vi "OSF Upload File.vi"(6 "Append to\nLab Notebook":bool, 7 "timeout":dbl=60.0 format="%#_6ps", 8 "error in":errorcluster, 9 "Token":string, 10 "Node":string, 11 "File name":path=path "C:/Data/April_2019/042419/sp0006_042419.tdms") -> (0 "error out":errorcluster)   [LabVIEW 2021]
uses:
  <vilib>/httpClient/LabVIEWHTTPClient.lvlib
  <vilib>/httpClient/PUTFile.vi
  <vilib>/httpClient/PUTBuffer.vi
  <vilib>/Utility/TDMS File Viewer/NI_TDMS File Viewer.lvlib
panel:
  in  "View":bool
  out "Status":string
  in  "Upload":bool
  in  "Stop Button":bool
  in  "Export Type":enum16{"Text", "Markdown"}(ring)=enum."Markdown"
  out "Elapsed time":dbl format="%#_6ps"
  out "body 2":string
  out "body":string
  in  "OSF API URL":string="https://api.osf.io/v2/"
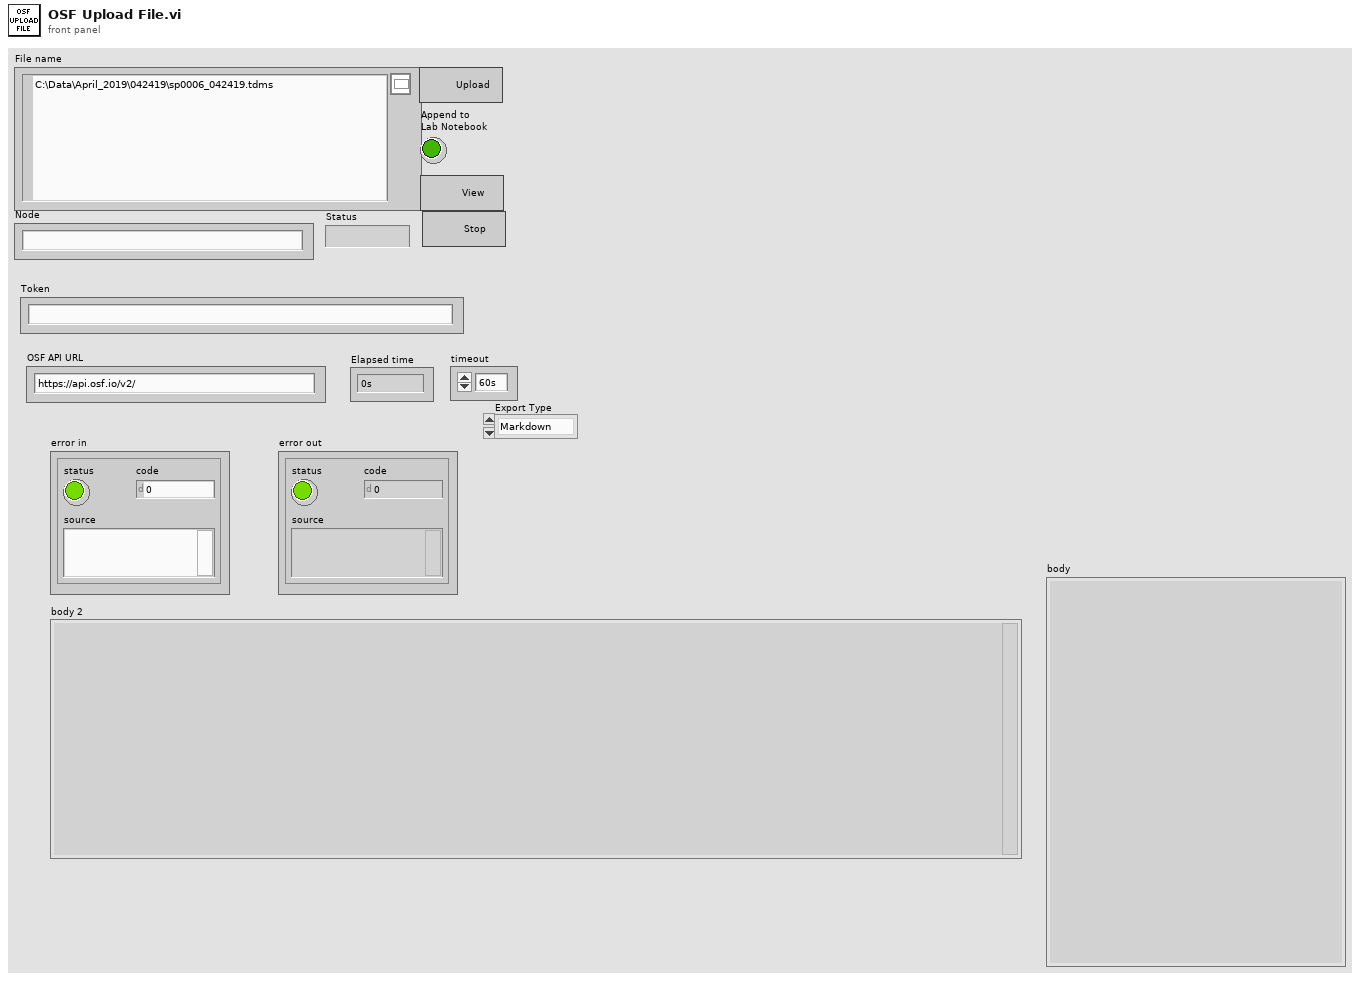
[diagram p1: front panel]
types:
  T1 = typedef "LabVIEWHTTPClient.lvlib/ClientHandle.ctl" = refnum<k1>
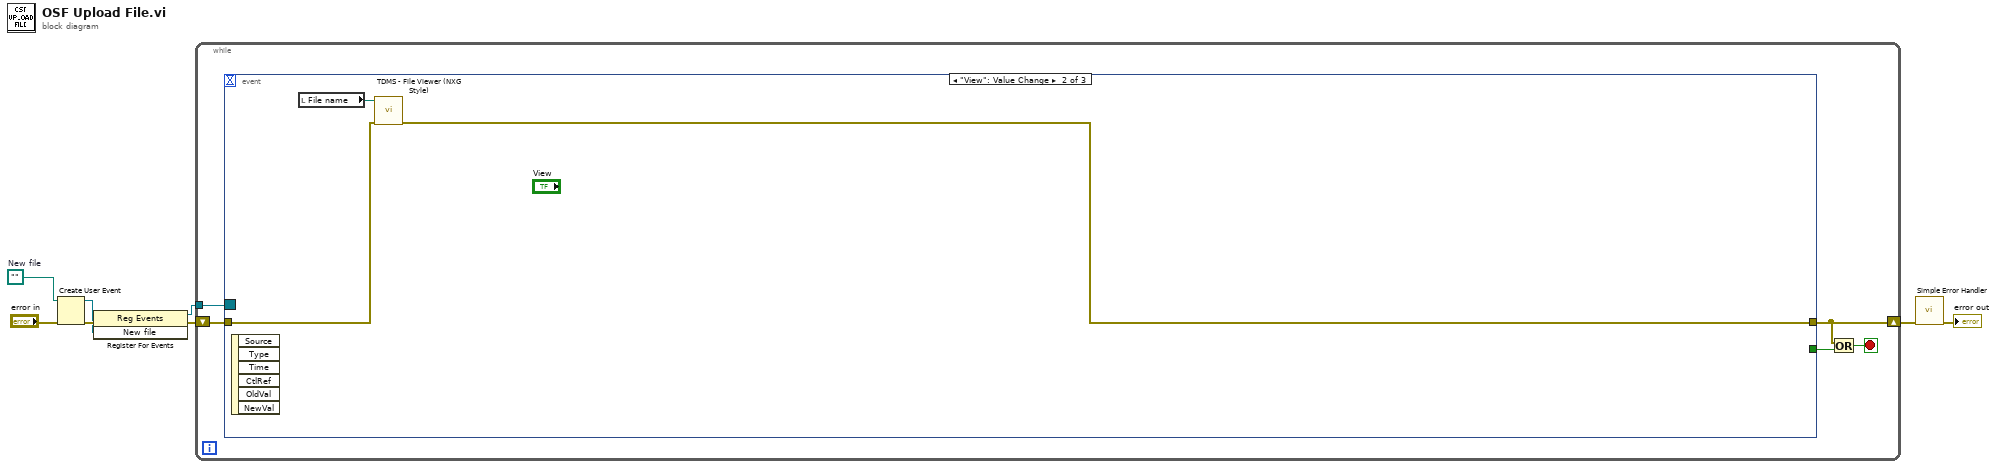
[diagram p0: block diagram]
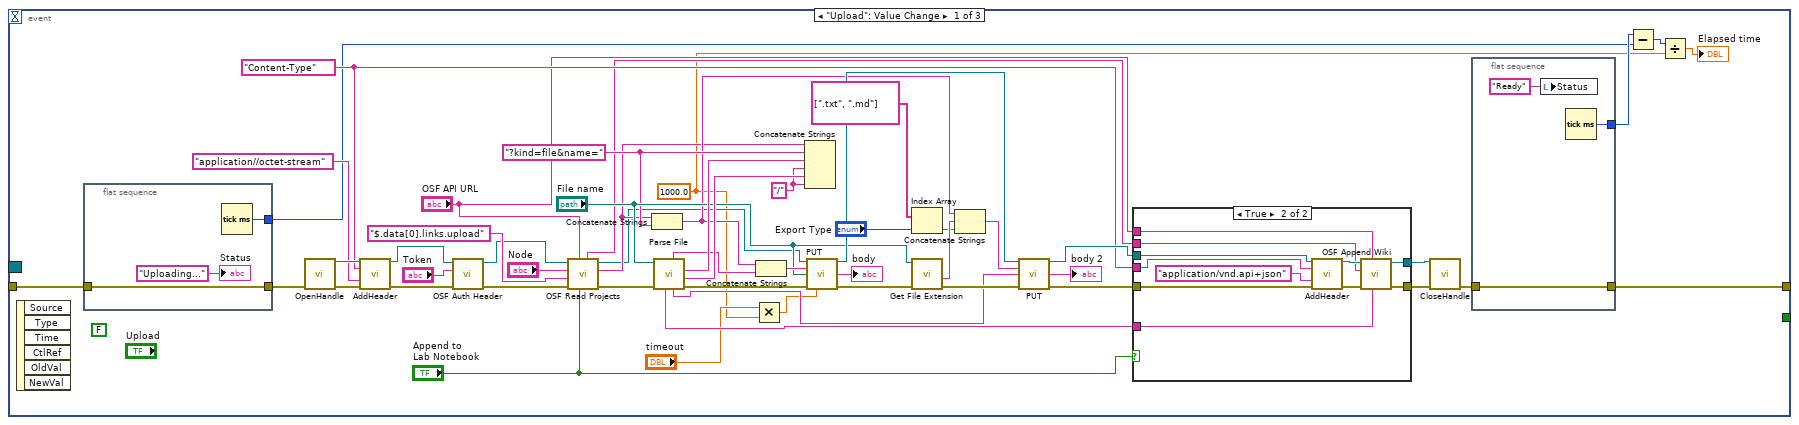
[diagram p2: hidden frame]
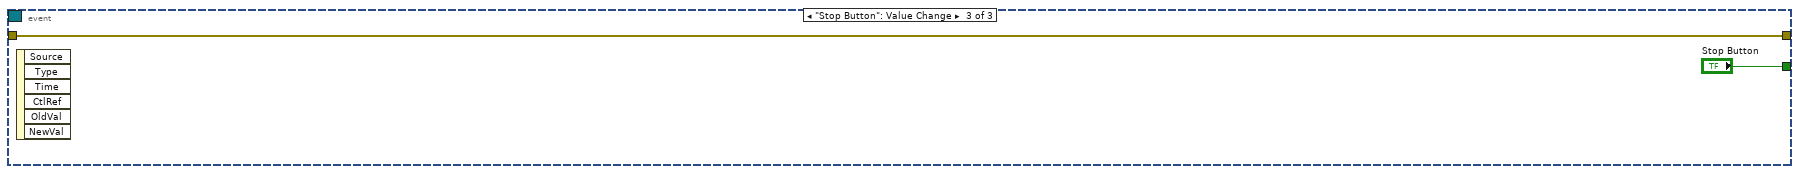
[diagram p4: hidden frame]
diagram:
  w3 = path ""  # New file
  n1 = Create User Event(user event datatype=w3, error in="error in") -> (user event=w1:refnum<user-event>, error out=w4:errorcluster)
  n2 = register-events(error in=w4, w1) -> (reference out=w5:refnum<event-registration>, error out=w6:errorcluster)  [unwired: 1 in]
  n3 = while {
    shift-right: [w10] -> w7
    shift-left: w6 -> [w13]
    tunnel: w5 -> [w9]
    stop <- w11 stop-if-true
    n4 = event shown="[1] \"View\": Value Change" {
      selector: w9 -> [_ _ _]
      dyn-events: _ -> [_ _ _]
      timeout: _ -> [_ _ _]
      tunnel: w13 -> [w25 w87 w89]
      tunnel: [w22 w86 w89] -> w10
      tunnel: [_ _ "Stop Button"] -> w12
      event "Upload": Value Change {
        (unwired) FALSE ("Top Button")
        w17 = 1000.0 ("y")
        w57 = "/" ("string")
        w46 = "?kind=file&name="
        w38 = "Content-Type" ("header")
        n5 = event-data() -> ()  [unwired: 1 in, 6 out]
        n6 = flat-sequence {
          tunnel: w25 -> [w72]
          tunnel: [w72] -> w24
          tunnel: [w71] -> w20
          frame #0 {
            n7 = Tick Count (ms)() -> (millisecond timer value=w71:u32)
            "Status" <- "Uploading..." ("Status")
          }
        }
        n8 = call <vilib>:"OpenHandle.vi"("error in (no error)"=w24) -> ("client handle out"=w66:T1, "error out"=w65:errorcluster)  [unwired: 13 in]
        n9 = call <vilib>:"AddHeader.vi"("client handle"=w66, "header"=w38, "value"="application//octet-stream", "error in (no error)"=w65) -> ("client handle out"=w61:T1, "error out"=w33:errorcluster)  [unwired: 10 in]
        n10 = call "OSF Auth Header.vi"("error in"=w33, "Token"="Token", "client handle"=w61) -> ("error out"=w30:errorcluster, "client handle out"=w31:T1)  [unwired: 7 in]
        n11 = call "OSF Read Projects.vi"("Read wikis"="Append to\nLab Notebook", "OSF API URL"="OSF API URL", "error in"=w30, "$Path or Item Name"="$.data[0].links.upload", "node"="Node", "client handle"=w31) -> ("error out"=w29:errorcluster, "Upload link"=w36:string, "client handle out"=w32:T1, "Wiki ID"=w35:string)  [unwired: 2 out]
        n12 = Concatenate Strings(w36, w46) -> (w45:string)
        n13 = call "Parse File.vi"("error in"=w29, "File name"="File name") -> ("error out"=w56:errorcluster, "Dir 2"=w58:string, "Dir 1"=w59:string, "metadata"=w41:string, "File name"=w42:string, "Lab notebook entry"=w28:string)  [unwired: 2 in, 2 out]
        n14 = Multiply(x="timeout", y=w17) -> (x*y=w26:dbl)
        n15 = Concatenate Strings(w45, w42) -> (w54:string)
        n16 = Concatenate Strings(w36, w46, w59, w57, w58, w57) -> ()  [unwired: 1 out]
        n17 = call-poly <vilib>:"PUT.vi"("client handle"=w32, "url"=w54, "file"="File name", "error in (no error)"=w56, "timeout (10000)"=w26) -> ("client handle out"=w55:T1, "body"=→"body":string, "error out"=w49:errorcluster)  [unwired: 7 in, 1 out]
        n18 = Index Array(array=string[] [".txt", ".md"], index="Export Type") -> (element=w16:string)
        n19 = call <vilib>:"Get File Extension.vi"("error in (no error)"=w49, "file"="File name") -> ("error out"=w48:errorcluster, "filename without extension"=w52:string)  [unwired: 5 in, 3 out]
        n20 = Concatenate Strings(w45, w52, w16) -> (w51:string)
        n21 = call-poly <vilib>:"PUT.vi"("client handle"=w55, "url"=w51, "buffer"=w41, "error in (no error)"=w48) -> ("client handle out"=w39:T1, "body"=→"body 2":string, "error out"=w40:errorcluster)  [unwired: 8 in, 1 out]
        n22 = case shown="True" "Append to\nLab Notebook" {
          tunnel: [w73 w85] -> w44
          tunnel: [w74 w84] -> w43
          tunnel: w28 -> [_ w83]
          tunnel: w40 -> [w74 w82]
          tunnel: w39 -> [w73 w80]
          tunnel: w38 -> [_ w78]
          tunnel: "OSF API URL" -> [_ w76]
          tunnel: w35 -> [_ w75]
          frame False {
          }
          frame True {
            n23 = call <vilib>:"AddHeader.vi"("client handle"=w80, "header"=w78, "value"="application/vnd.api+json", "error in (no error)"=w82) -> ("client handle out"=w79:T1, "error out"=w81:errorcluster)  [unwired: 10 in]
            n24 = call "OSF Append Wiki.vi"("content"=w83, "OSF API URL"=w76, "error in"=w81, "Wiki  ID"=w75, "client handle"=w79) -> ("error out"=w84:errorcluster, "client handle out"=w85:T1)  [unwired: 4 in, 1 out]
          }
        }
        n25 = call <vilib>:"CloseHandle.vi"("client handle"=w44, "error in (no error)"=w43) -> ("error out"=w23:errorcluster)  [unwired: 13 in]
        n26 = flat-sequence {
          tunnel: w23 -> [w69]
          tunnel: [w69] -> w22
          tunnel: [w68] -> w21
          frame #0 {
            n27 = local write "Status"("Ready" ("Status")) -> ()
            n28 = Tick Count (ms)() -> (millisecond timer value=w68:u32)
          }
        }
        n29 = Subtract(x=w21, y=w20) -> (x-y=w18:u32)
        n30 = Divide(x=w18, y=w17) -> (x/y=→"Elapsed time":dbl)
      }
      event "View": Value Change {
        n31 = event-data() -> ()  [unwired: 1 in, 6 out]
        n32 = local read "File name"() -> (w88:path)
        n33 = call <vilib>:"TDMS - File Viewer (NXG Style).vi"("error in"=w87, "file in"=w88) -> ("error out"=w86:errorcluster)  [unwired: 8 in, 1 out]
      }
      event "Stop Button": Value Change {
        n34 = event-data() -> ()  [unwired: 1 in, 6 out]
      }
    }
    n35 = Or(x=w10, y=w12) -> (x .or. y?=w11:bool)
  }
  n36 = call <vilib>:"Simple Error Handler.vi"("error in (no error)"=w7) -> ("error out"=→"error out":errorcluster)  [unwired: 4 in, 4 out]
